vi "ACIR.vi"(8 "error in":errorcluster, 9 "Setting":T1={"Freq"=1000.0, "Range"=enum."10m Ohm", "Measurements"=enum."OCV"} {"Freq" min=0.1 max=1050.0 step=0.01 format="%_5e"}, 10 "ACIR Ref":string, 11 "Analog In":refnum<class "Analog In.lvclass">) -> (0 "error out":errorcluster, 2 "Measurements":dbl[](array[numeric]), 3 "Analog In":refnum<class "Analog In.lvclass">)   [LabVIEW 2019, in "Code Modules.lvlib"]
uses:
  Code Modules.lvlib
  PPLs/Hardware Abstraction.lvlibp/Harware Abstraction/Analog In/Analog In.lvclass
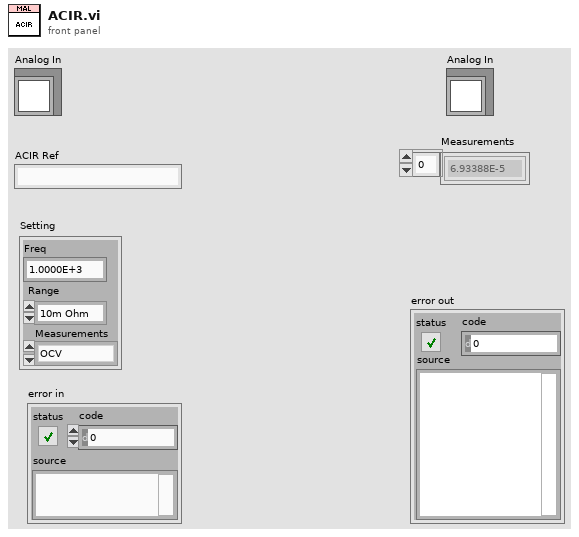
[diagram p1: front panel]
types:
  T1 = cluster{"Freq":dbl, "Range":enum16{"3m Ohm", "10m Ohm", "100m Ohm"}, "Measurements":enum16{"Impedence", "Phase Angle", "OCV"}}
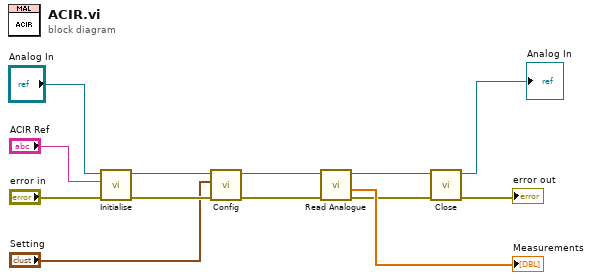
[diagram p0: block diagram]
diagram:
  n1 = call-dynamic "Initialise.vi"("error in (no error)"="error in", "Instrument Ref"="ACIR Ref", "Instrument in"="Analog In") -> ("error out"=w10:errorcluster, "Instrument out"=w9:refnum<class "Analog In.lvclass">)  [unwired: 7 in]
  n2 = call-dynamic "Config.vi"("error in (no error)"=w10, "Setting"="Setting", "Analog In in"=w9) -> ("error out"=w6:errorcluster, "Analog In out"=w7:refnum<class "Analog In.lvclass">)  [unwired: 7 in]
  n3 = call-dynamic "Read Analogue.vi"("error in (no error)"=w6, "PS in"=w7) -> ("error out"=w3:errorcluster, "Measurements"=→"Measurements":dbl[], "PS out"=w4:refnum<class "Analog In.lvclass">)  [unwired: 6 in, 1 out]
  n4 = call-dynamic "Close.vi"("error in (no error)"=w3, "Instrument in"=w4) -> ("error out"=→"error out":errorcluster, "Instrument out"=→"Analog In":refnum<class "Analog In.lvclass">)  [unwired: 8 in]
